vi "eReadNames Loop.vi"() -> (0 "error out":errorcluster)   [LabVIEW 2020]
panel:
  out "Iteration":u32
  in  "stop":bool
  in  "Interval [ms]":i32=500
  in  "Read Names":string[](array[string])=["AIN0", "FIO2"]
  out "Error String":string
  out "ConnectionType Out":i32
  out "DeviceType Out":i32
  in  "Identifier":string="LJM_idANY"
  in  "ConnectionType":string="LJM_ctANY"
  in  "DeviceType":string="LJM_dtANY"
  out "Read Values":dbl[](array[numeric]) format="%.6f"
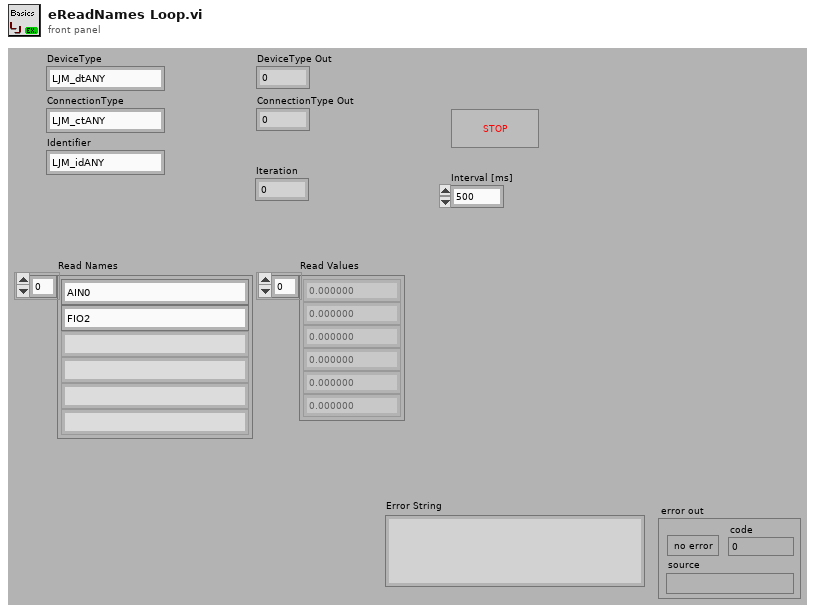
[diagram p1: front panel]
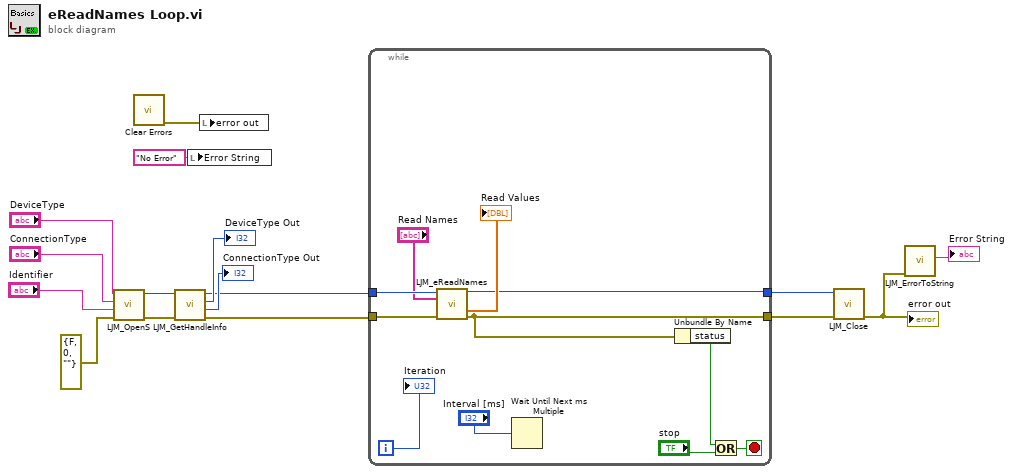
[diagram p0: block diagram]
diagram:
  n1 = call "LJM_OpenS.vi"("error in"=errorcluster {"status"=FALSE, "code"=0, "source"=""}, "Identifier"="Identifier", "ConnectionType"="ConnectionType", "DeviceType"="DeviceType") -> ("error out"=w16:errorcluster, "Handle"=w15:i32)  [unwired: 6 in]
  n2 = call <vilib>:"Clear Errors.vi"() -> ("error out"=w3:errorcluster)  [unwired: 6 in, 1 out]
  n3 = call "LJM_GetHandleInfo.vi"("error in"=w16, "Handle In"=w15) -> ("error out"=w4:errorcluster, "ConnectionType"=→"ConnectionType Out":i32, "DeviceType"=→"DeviceType Out":i32, "Handle Out"=w5:i32)  [unwired: 2 in, 4 out]
  n4 = local write "Error String"("No Error" ("Error String")) -> ()
  n5 = local write "error out"(w3) -> ()
  n6 = while {
    tunnel: w4 -> [w27]
    tunnel: [w18] -> w7
    tunnel: w5 -> [w26]
    tunnel: [w19] -> w6
    i -> [w17]
    stop <- w23 stop-if-true
    n7 = call "LJM_eReadNames.vi"("Handle In"=w26, "aNames"="Read Names", "error in"=w27) -> ("Handle Out"=w19:i32, "aValuesOut"=→"Read Values":dbl[], "error out"=w18:errorcluster)  [unwired: 9 in, 1 out]
    n8 = Wait Until Next ms Multiple(millisecond multiple="Interval [ms]") -> ()  [unwired: 1 out]
    n9 = Unbundle By Name(w18) -> ("status"=w22:bool)
    n10 = Or(x=w22, y="stop") -> (x .or. y?=w23:bool)
    "Iteration" <- w17
  }
  n11 = call "LJM_Close.vi"("error in"=w7, "Handle"=w6) -> ("error out"=w9:errorcluster)  [unwired: 9 in]
  "error out" <- w9
  n12 = call "LJM_ErrorToString.vi"("error in"=w9) -> ("String"=→"Error String":string)  [unwired: 10 in]
